vi "LVAPT-GIT-SwitchToDailyBranch.vi"(11 "path":path) -> ()   [LabVIEW 2019]
uses:
  <vilib>/Hampel Software Engineering/Git API/Git API/GIT-api.lvclass/GIT-api.ctl
  <vilib>/Hampel Software Engineering/Git API/Git API/Accessors/GIT-Set Working Dir.vi
  <vilib>/Hampel Software Engineering/Git API/Git API/GIT-api.lvclass
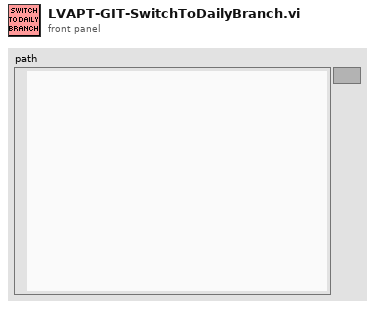
[diagram p1: front panel]
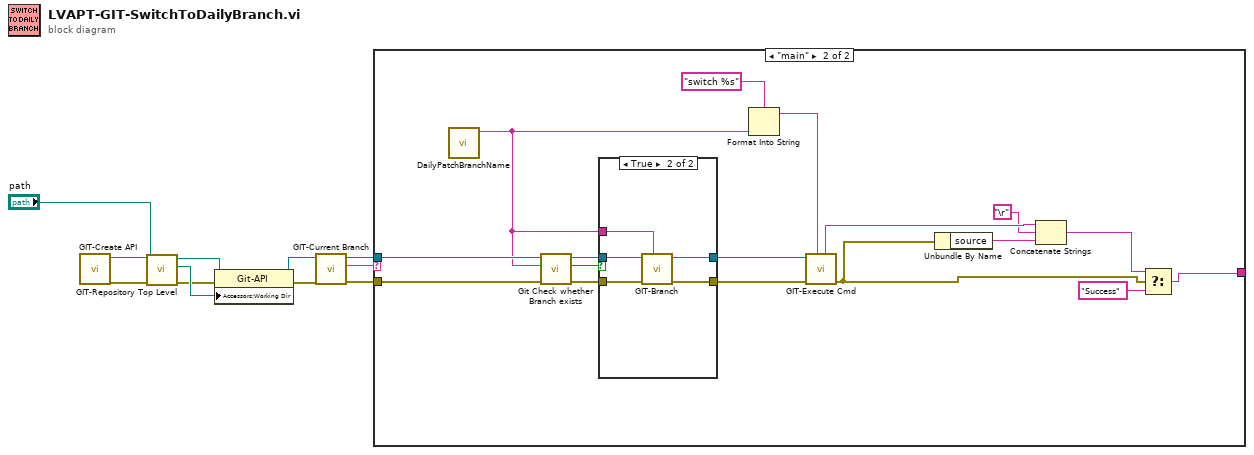
[diagram p0: block diagram]
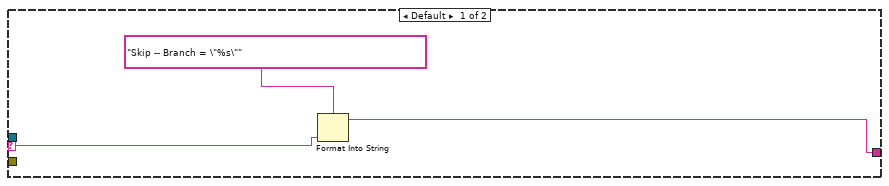
[diagram p2: hidden frame]
diagram:
  n1 = call <vilib>:"GIT-Create API.vi"() -> ("error out"=w7:errorcluster, "git-api out"=w6:refnum<class "GIT-api.lvclass">)  [unwired: 10 in]
  n2 = call <vilib>:"GIT-Repository Top Level.vi"("error in"=w7, "Current Path"="path", "git-api in"=w6) -> ("error out"=w1:errorcluster, "Repo Top Level Path"=w3:path, "git-api out"=w2:refnum<class "GIT-api.lvclass">)  [unwired: 6 in]
  n3 = property class="Git-API"(reference=w2, error in=w1, "Accessors:Working Dir"=w3) -> (reference out=w4:refnum<class "GIT-api.lvclass">, error out=w5:errorcluster)
  n4 = call <vilib>:"GIT-Current Branch.vi"("error in"=w5, "git-api in"=w4) -> ("error out"=w9:errorcluster, "current branch"=w8:string, "git-api out"=w10:refnum<class "GIT-api.lvclass">)  [unwired: 7 in]
  n5 = case shown="\"main\"" w8 {
    selector: w8 -> [w13 _]
    tunnel: w9 -> [_ w26]
    tunnel: w10 -> [_ w27]
    tunnel: [w12 w15] -> _
    frame Default {
      n6 = Format Into String(format string="Skip -- Branch = \"%s\"" ("f"), w13) -> (resulting string=w12:string)  [unwired: 2 in, 1 out]
    }
    frame "main" {
      n7 = call "DailyPatchBranchName.vi"() -> ("DailyPatchBranchName"=w23:string)  [unwired: 11 in]
      n8 = call "Git Check whether Branch exists.vi"("error in (no error)"=w26, "DailyPatchBranchName"=w23, "GIT-api in"=w27) -> ("error out"=w25:errorcluster, "Boolean"=w22:bool, "GIT-api out"=w24:refnum<class "GIT-api.lvclass">)  [unwired: 6 in]
      n9 = case shown="True" w22 {
        tunnel: [w33 w38] -> w31
        tunnel: [w32 w37] -> w30
        tunnel: w25 -> [w32 w36]
        tunnel: w24 -> [w33 w35]
        tunnel: w23 -> [_ w34]
        frame False {
        }
        frame True {
          n10 = call <vilib>:"GIT-Branch.vi"("param"=w34, "error in"=w36, "git-api in"=w35) -> ("error out"=w37:errorcluster, "git-api out"=w38:refnum<class "GIT-api.lvclass">)  [unwired: 6 in, 1 out]
        }
      }
      n11 = Format Into String(format string="switch %s", w23) -> (resulting string=w28:string)  [unwired: 2 in, 1 out]
      n12 = call <vilib>:"GIT-Execute Cmd.vi"("Command"=w28, "error in"=w30, "Git-API in"=w31) -> ("error out"=w17:errorcluster, "std out"=w19:string)  [unwired: 6 in, 1 out]
      n13 = Unbundle By Name(w17) -> ("source"=w20:string)
      n14 = Concatenate Strings(w19, "\r", w20) -> (w21:string)
      n15 = Select(t=w21, s=w17, f="Success") -> (s? t:f=w15:string)
    }
  }
